vi "Set Channel Blocks.vi"(10 "channel blocks":T1[](array[typedef]) {"buffer offset" format="%d bytes"}, 11 "Transfer Configuration in":refnum<class "Transfer Configuration.lvclass">) -> (3 "Transfer Configuration out":refnum<class "Transfer Configuration.lvclass">)   [LabVIEW 2017, in "Data Sharing Framework Core.lvlib" / "Data Sharing Framework Engine.lvlib" / "Transfer Configuration.lvclass"]
uses:
  Transfer Configuration.lvclass
  Type Definitions/DSF Runtime Channel Block.ctl
  Configuration/1.0.0/Public/Controls/DSF Data Type.ctl
  Transfer Configuration.lvclass/Transfer Configuration.ctl
  Data Sharing Framework Engine.lvlib
  Configuration/1.0.0/Data Sharing Framework Configuration.lvlib
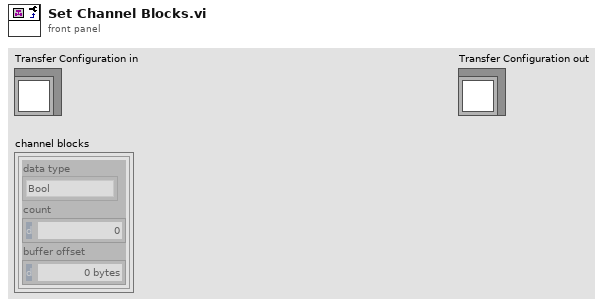
[diagram p1: front panel]
types:
  T1 = typedef "Data Sharing Framework Core.lvlib/Data Sharing Framework Engine.lvlib/DSF Runtime Channel Block.ctl" = cluster{"data type":T2, "count":u64, "buffer offset":u64}
  T2 = typedef "Data Sharing Framework Core.lvlib/Data Sharing Framework Configuration.lvlib/DSF Data Type.ctl" = enum8{"Bool", "SGL", "DBL", "I8", "I16", "I32", "I64", "U8", "U16", "U32", "U64"}
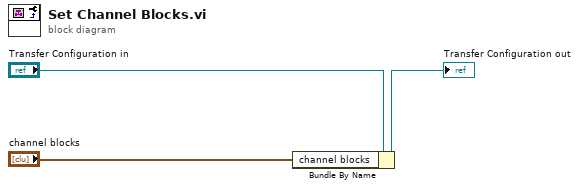
[diagram p0: block diagram]
diagram:
  n1 = Bundle By Name(cluster="Transfer Configuration in", "channel blocks"="channel blocks") -> (→"Transfer Configuration out":refnum<class "Transfer Configuration.lvclass">)
